vi "EndevoGOOP400Provider_Configuration.vi"(1 "ClassRef/ClassPath(If empty Configuration default will be modified)":variant, 5 "Error In":errorcluster) -> (15 "SelectedWireStyleIndex":i32, 19 "Error Out":errorcluster)   [LabVIEW 2020]
uses:
  <resource>/Framework/Providers/Open_GDS/ClassProviders/Common/LvIcon_class/GDSLvIcon_ColorControl.ctl
  <resource>/Framework/Providers/Open_GDS/SubVIs/GOOP_WirePattern.ctl
  <resource>/Framework/Providers/Open_GDS/ClassProviders/Common/ScriptingFunctions/Scripting_ConnectorPanePatternType.ctl
  <resource>/Framework/Providers/Open_GDS/ClassProviders/Provider_BaseClassInterface/BaseProvider_SubVIs/BaseProvider_WireStyleType.ctl
  <resource>/Framework/Providers/Open_GDS/SubVIs/GOOP_WireConfigurationType.ctl
  <resource>/Framework/Providers/Open_GDS/ClassProviders/Common/CommonVIs/CommonVIs_ClassIconSelection_Action.ctl
  <resource>/Framework/Providers/Open_GDS/ClassProviders/Provider_BaseClassInterface/BaseProvider_SubVIs/BaseProvider_FileNamingOption.ctl
  <resource>/Framework/Providers/Open_GDS/ClassProviders/Provider_EndevoGOOP400/GOOP400_SubVIs/GOOP400_Options.ctl
panel:
  in  "_CleanUpBDForPropertyMethods":bool caption="Use flat folder structure for new classes"
  in  "File naming option":T1(ring)
  out "IconSelection":picture
  in  "_FlatFolderStructure":bool caption="Use flat folder structure for new classes"
  in  "WireStyleList":T2[](array[typedef])
  in  "DiscardChanges":bool
  in  "Update/AddWireStyle":bool
  in  "DeleteWireStyle":bool
  in  "Down":bool
  in  "Up":bool
  in  "WireStyleName":string caption="Selected Wire Style Name"
  out "ProductPicture":picture
  out "Icon":picture
  in  "_Dice":cluster{"Boolean 2":bool, "Dice 2":bool}
  in  "_DefaultConnectorPanePattern":T3 caption="Default Connector Pane Pattern" items=["4x4x4", "5x6x5", "6x8x6"]
  in  "_HelpDefaultConfiguration":bool
  in  "_Help":bool
  out "_ClassItemIconApperance":string caption="Class Item Icon Appearance"
  out "_WireApperance":string
  in  "_SetToDefaultForAllClasses":bool caption="Set this to default\nfor all future classes"
  in  "_Cancel":bool
  out "_Preview":picture caption="Preview"
  in  "_Icon":u16(ring) caption="Icon" items=["BlueFull", "BlueFrame", "InterfaceBlue", "BlueCircle", "BrownFull", "BrownFrame", "InterfaceBrown", "BrownCircle", "BurgundyFull", "BurgundyFrame", "InterfaceBurgundy", "BurgundyCircle", "CyanFull", "CyanFrame", "InterfaceCyan", "CyanCircle", "DarkBlueFull", "DarkBlueFrame", "InterfaceDarkBlue", "DarkBlueCircle", "ForestGreenFull", "ForestGreenFrame", "InterfaceForestGreen", "ForestGreenCircle", "GrayFull", "GrayFrame", "InterfaceGray", "GrayCircle", "GreenFull", "GreenFrame", "InterfaceGreen", "GreenCircle", "LightGreenFull", "LightGreenFrame", "InterfaceLightGreen", "LightGreenCircle", "LightRedFull", "LightRedFrame", "InterfaceLightRed", "LightRedCircle", "PinkFull", "PinkFrame", "InterfacePink", "PinkCircle", "PurpleFull", "PurpleFrame", "InterfacePurple", "PurpleCircle", "RedFull", "RedFrame", "InterfaceRed", "RedCircle", "YellowFull", "YellowFrame", "InterfaceYellow", "YellowCircle"]
  in  "_TunnelsAndTerminalsColors":T4 caption="Tunnels and \nTerminals Colors"
  in  "_CenterColor2":T4 caption="Pattern Colors"
  in  "_CenterColor1":T4 caption="Pattern Colors"
  in  "_CenterPattern":T5 caption="Center pattern"
  in  "_EdgeColor":T4 caption="Edge color"
  in  "_CenterThickness":T6(ring) caption="Center thickness"
  in  "_EdgeThickness":T7(ring) caption="Edge thickness"
  out "Wire preview":picture
  in  "_Done":bool
  # "Wire Configuration"
  # "Wire Appearance"
  # "GOOP4 Options"
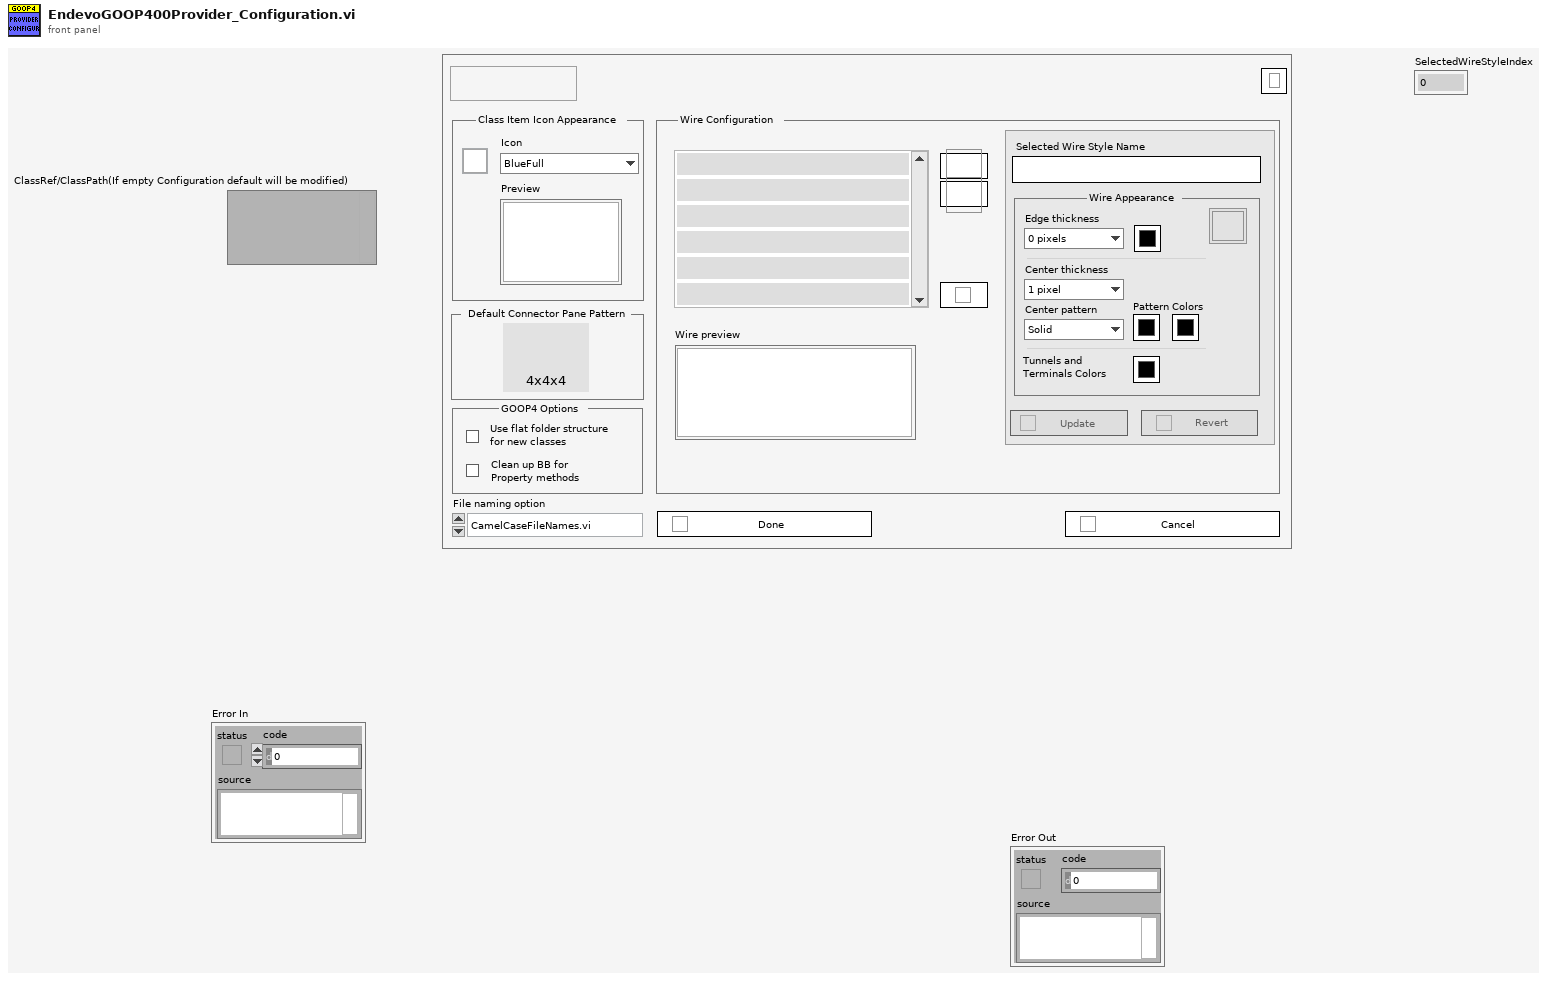
[diagram p1: front panel]
types:
  T1 = enum16{"CamelCaseFileNames.vi", "File Names With Spaces.vi", "File_Names_With_Underscores"}
  T2 = typedef "BaseProvider_WireStyleType.ctl" = cluster{"Boolean":bool, "Wire":picture, "Name":string, "Status":u16}
  T3 = typedef "Scripting_ConnectorPanePatternType.ctl" = u16
  T4 = typedef "GDSLvIcon_ColorControl.ctl" = cluster{"Decal":bool, "Color":u32}
  T5 = typedef "GOOP_WirePattern.ctl" = enum16{"Solid", "Large dash", "Small dash"}
  T6 = enum16{"1 pixel", "2 pixels", "3 pixels", "4 pixels", "5 pixels"}
  T7 = enum16{"0 pixels", "1 pixel", "2 pixels", "3 pixels"}
  T8 = typedef "GOOP_WireConfigurationType.ctl" = cluster{"Edge thickness":i32, "Edge color":u32, "Center thickness":i32, "Center pattern":T5, "CenterColor1":u32, "CenterColor2":u32, "Tunnels and terminals colors":u32}
  T9 = cluster{"FirstTime":bool, "ClassRef":refnum<vi>, "ClassRefCreated":bool, "CurrentWireStyle":T8, "DefaultIndex":i32, "SelectedWireStyleIndex":i32, "StartWireStyleIndex":i32}
  T10 = typedef "GOOP400_Options.ctl" = cluster{"FlatFolderStructure":bool, "CleanUpBDForPropertyMethods":bool}
  T11 = typedef "BaseProvider_FileNamingOption.ctl" = enum16{"CamelCase", "Space", "Underscore"}
  T12 = typedef "BaseProvider_IniFileSettings.ctl" = cluster{"ClassFolderSuffix":string, "InterfaceFolderSuffix":string, "InterfaceIcon":string, "FileNamingOption":T11, "DynamicDispatchStartValue":bool, "UseGetSetForPropertyNodeMethods":bool}
  T13 = typedef "GDSLvCLass_ClassSettingsType.ctl" = cluster{"ClassProviderName":string, "ClassTemplateUsed":string, "ClassTemplateVersion":string, "ClassDescription":string, "PlugIns":T14[], "ConnectorPanePattern":string}
  T14 = typedef "GDSLvClass_PlugIn.ctl" = cluster{"Type":T15, "ID":string, "Version":string, "Path":path, "Name":string, "Data":variant}
  T15 = typedef "GDSLvClass_PlugInTypes.ctl" = enum16{"DesignPattern", "MethodTypes"}
  T16 = cluster{"Foreground Color":u32, "Background Color":u32, "Fill Pattern":cluster{"Row 0":u8, "Row 1":u8, "Row 2":u8, "Row 3":u8, "Row 4":u8, "Row 5":u8, "Row 6":u8, "Row 7":u8}, "Width":i16, "Mode":enum16{"Copy", "Or", "Exclusive Or", "Bit Clear", "Not Copy", "Not Or", "Nor Exclusive Or", "Not Bit Clear"}, "Style":enum32{"Solid", "Dash", "Dot", "Dash Dot", "Dash Dot Dot"}, "Fill Rule":enum32{"Even Odd", "Winding"}, "End Caps":enum32{"Default", "Flat"}}[]
  T17 = enum8{"Enabled", "Disabled", "Disabled and Grayed Out"}
  T18 = typedef "imagedata.ctl" = cluster{"image type":i32, "image depth":i32, "image":u8[], "mask":u8[], "colors":u32[], "Rectangle":cluster{"left":i16, "top":i16, "right":i16, "bottom":i16}}
  T19 = typedef "CommonVIs_ClassIconSelection_Action.ctl" = enum16{"All", "Non Interface", "Only Interface"}
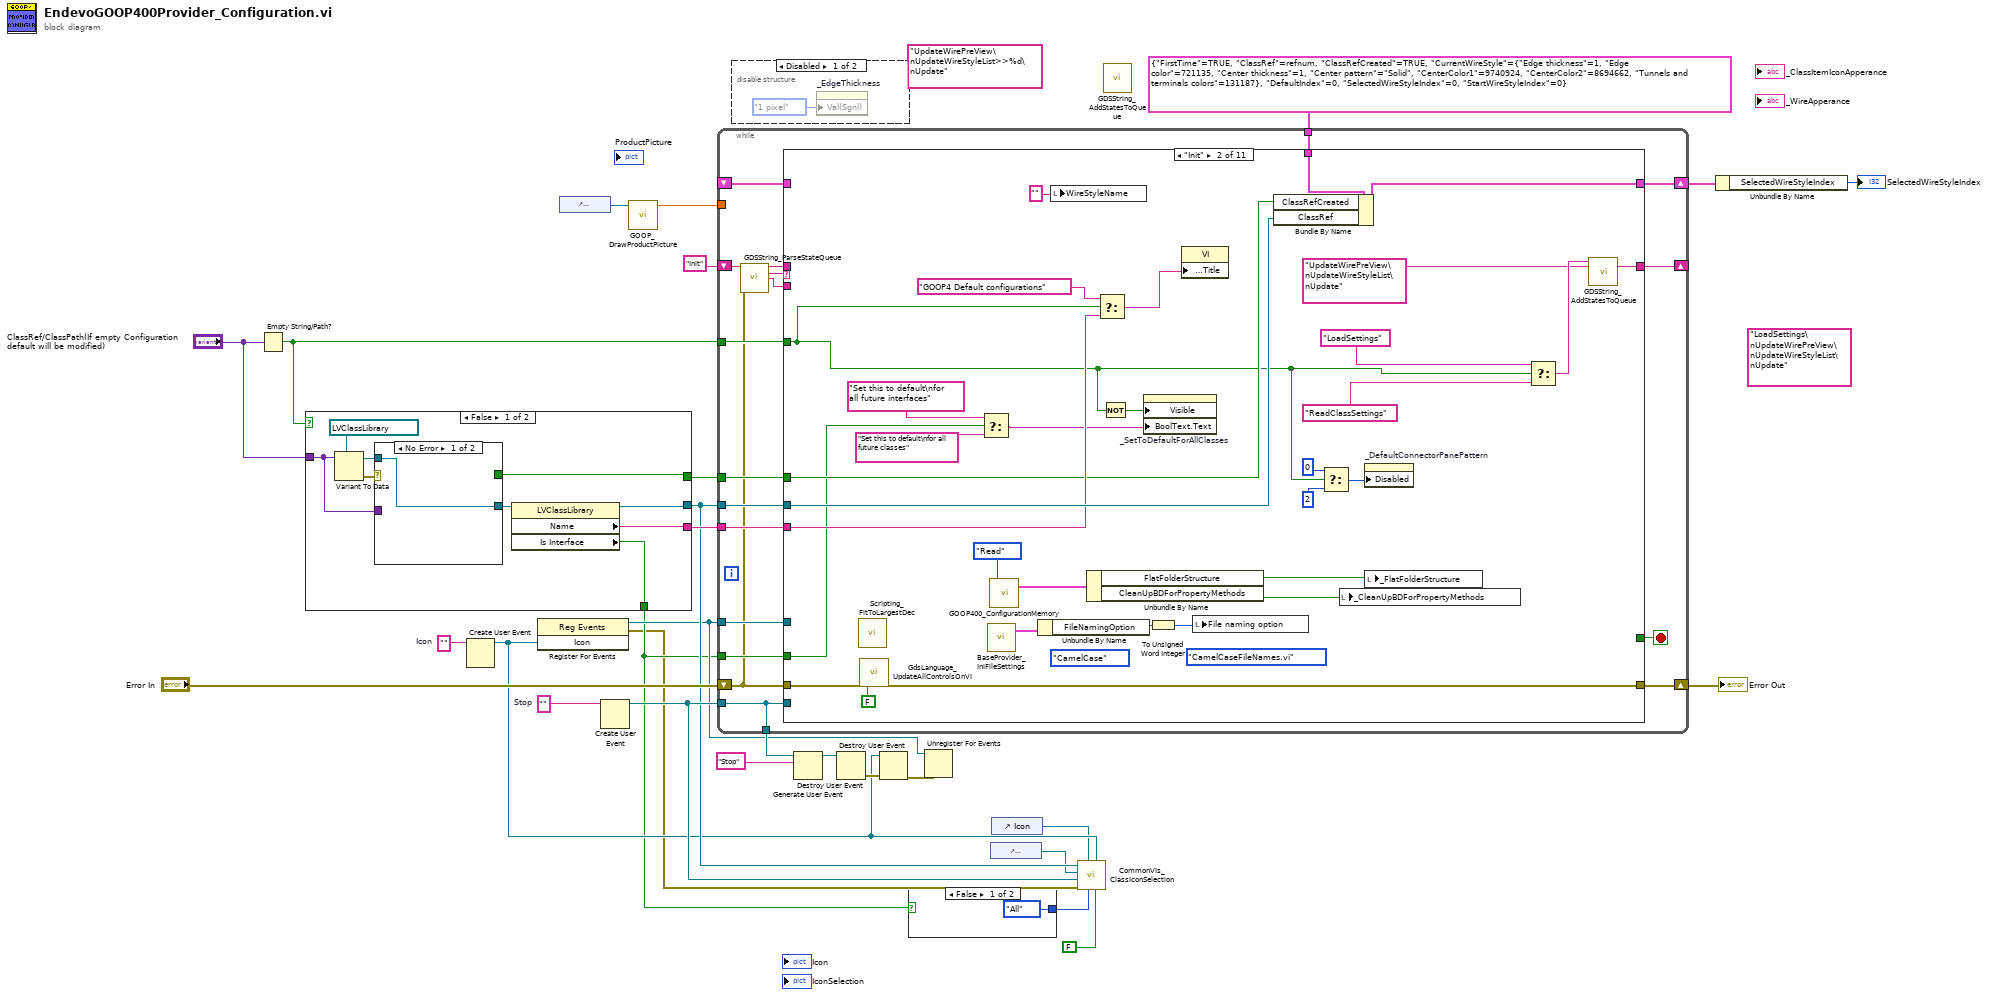
[diagram p0: block diagram]
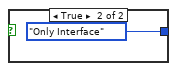
[diagram p2: hidden frame]
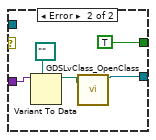
[diagram p4: hidden frame]
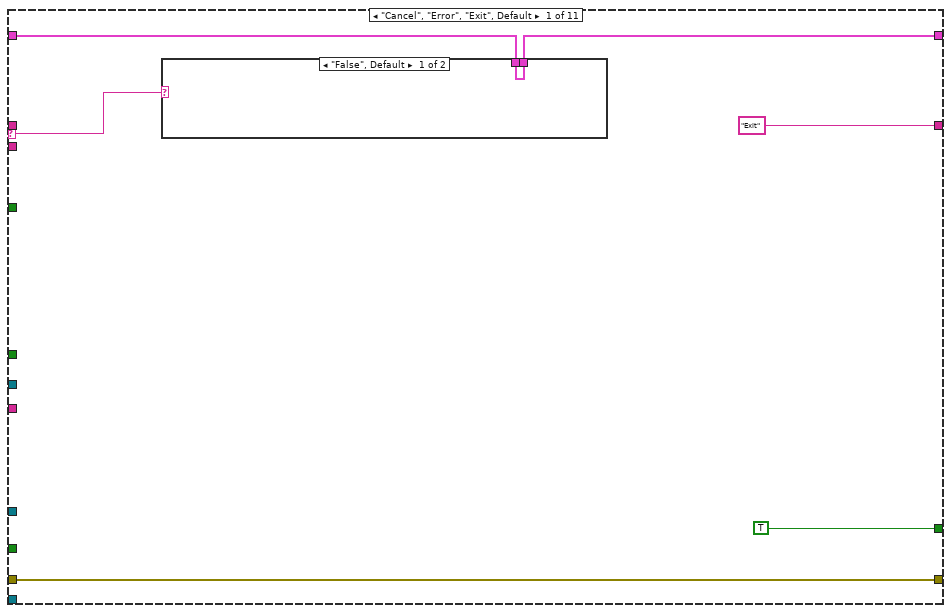
[diagram p6: hidden frame]
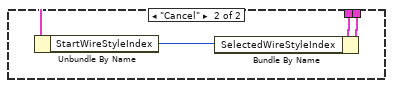
[diagram p7: hidden frame]
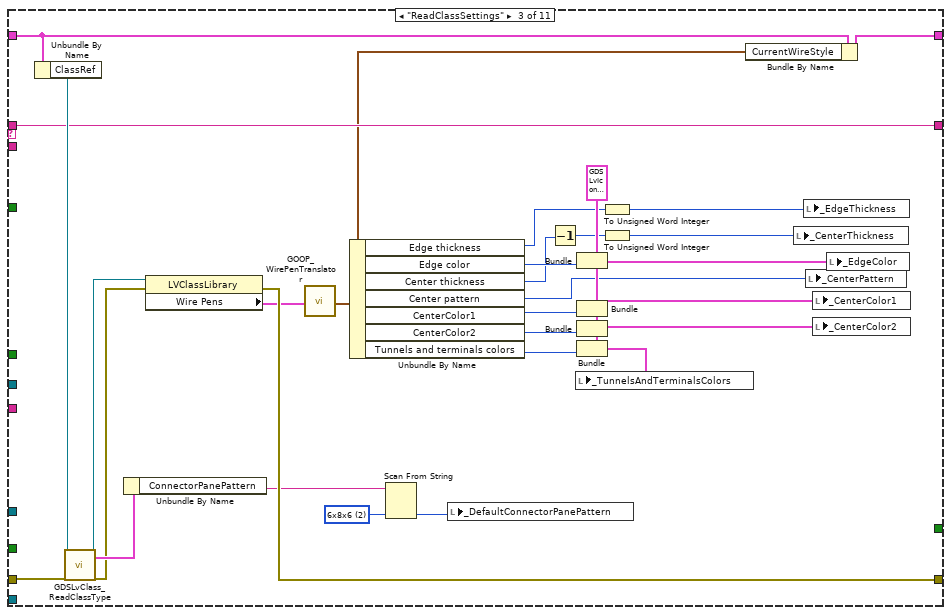
[diagram p8: hidden frame]
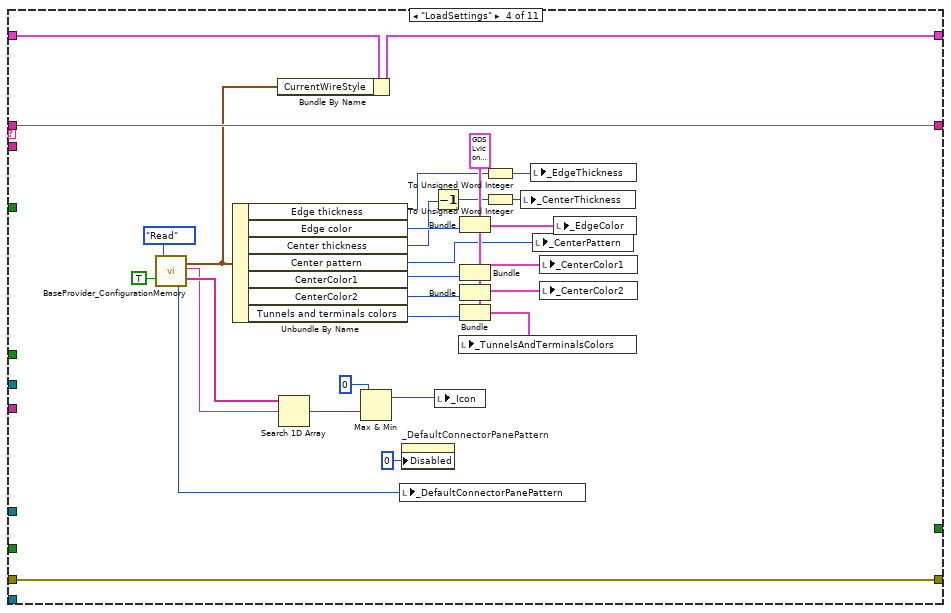
[diagram p9: hidden frame]
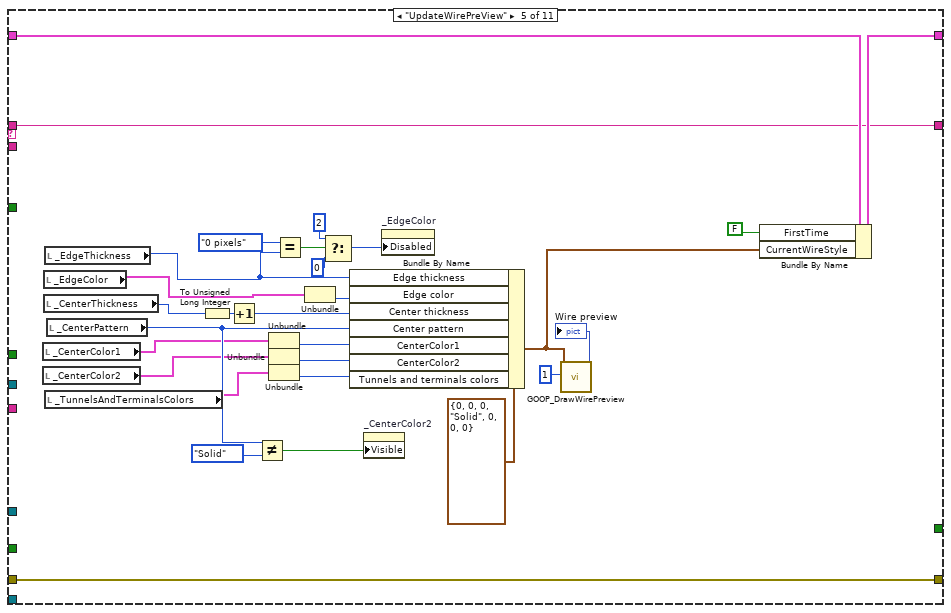
[diagram p10: hidden frame]
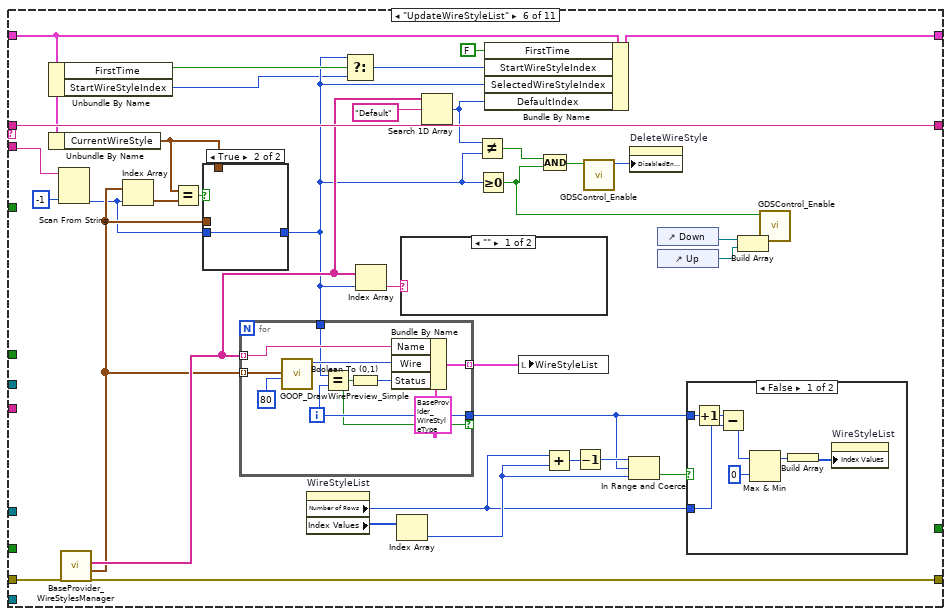
[diagram p11: hidden frame]
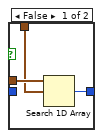
[diagram p12: hidden frame]
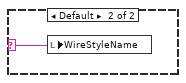
[diagram p14: hidden frame]
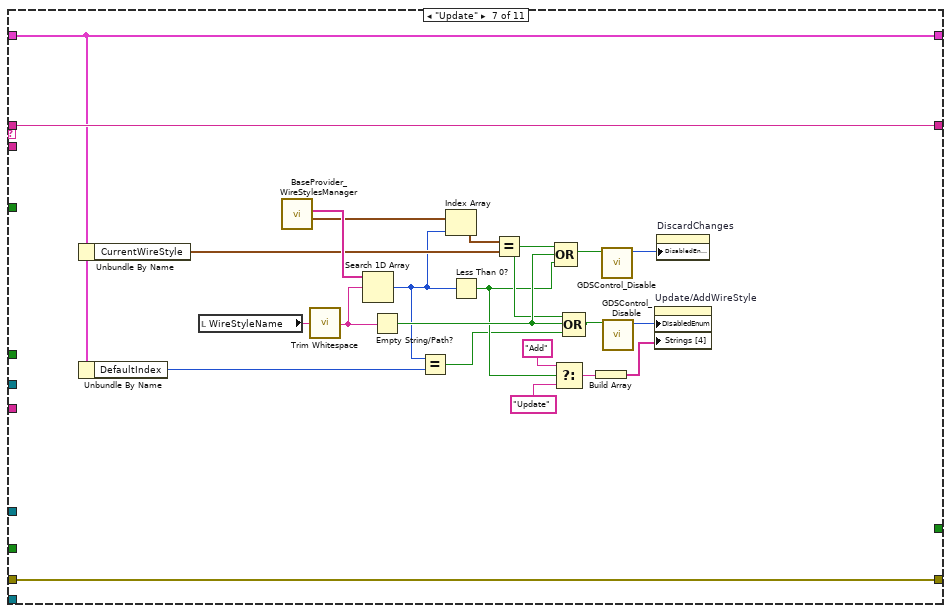
[diagram p15: hidden frame]
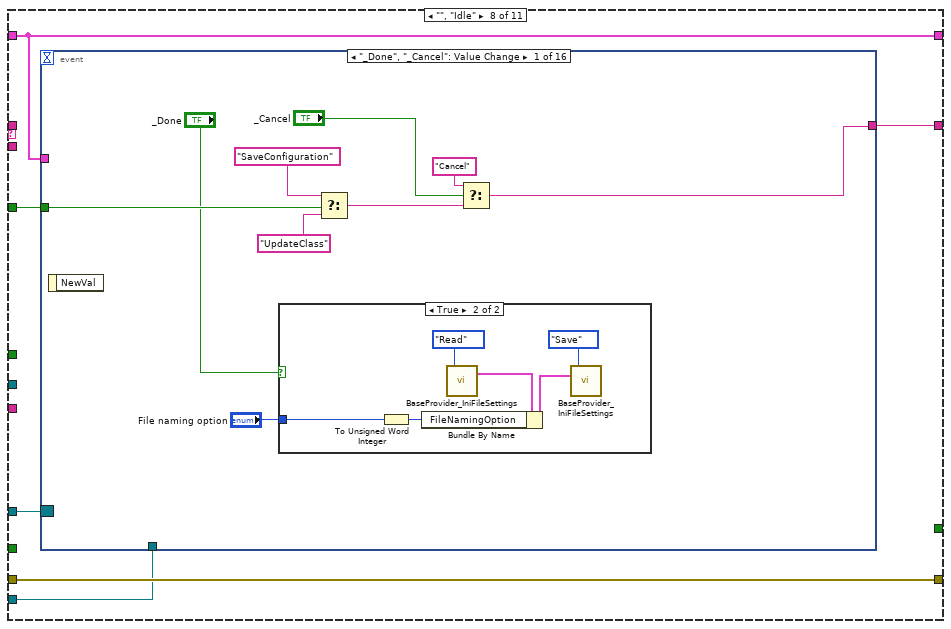
[diagram p16: hidden frame]
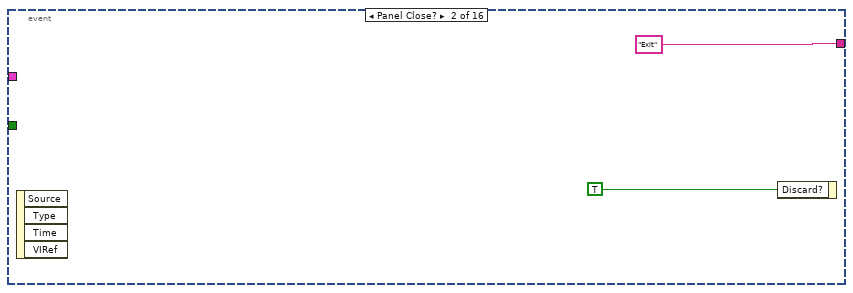
[diagram p18: hidden frame]
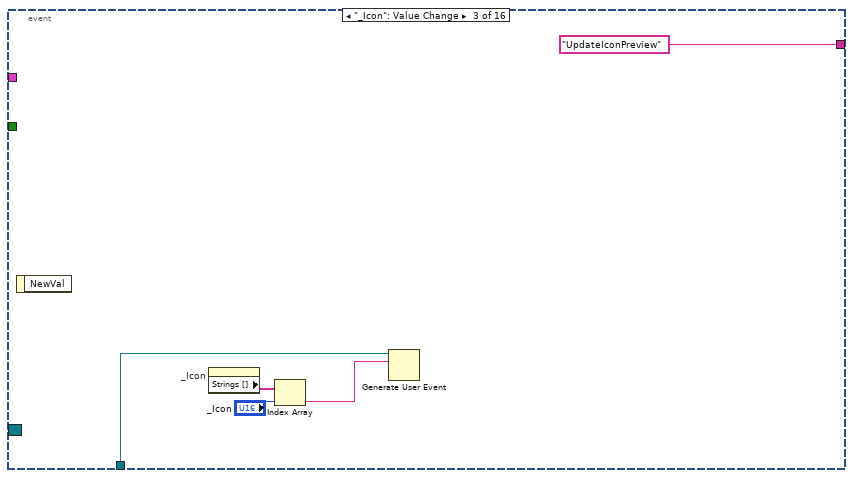
[diagram p19: hidden frame]
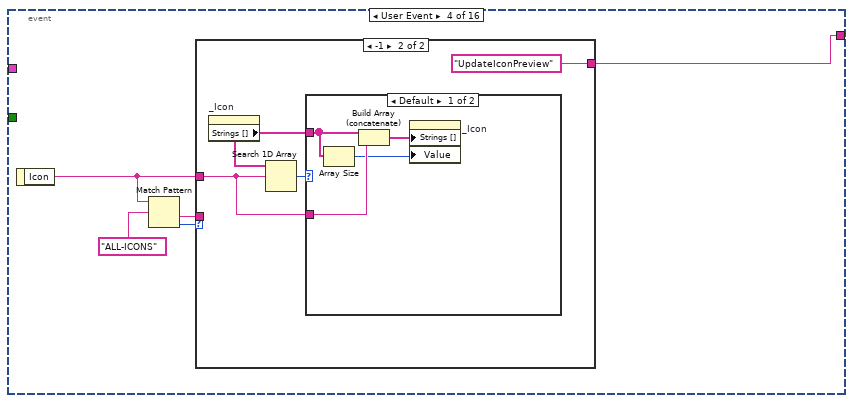
[diagram p20: hidden frame]
diagram:
  (unwired) "LoadSettings\nUpdateWirePreView\nUpdateWireStyleList\nUpdate"
  (unwired) "UpdateWirePreView\nUpdateWireStyleList>>%d\nUpdate"
  w16 = ""  # Icon
  w19 = ""  # Stop
  n1 = Empty String/Path?(string/path="ClassRef/ClassPath(If empty Configuration default will be modified)") -> (empty?=w21:bool)
  n2 = case shown="False" w21 {
    tunnel: "ClassRef/ClassPath(If empty Configuration default will be modified)" -> [w36 _]
    tunnel: [w32 _] -> w17
    tunnel: [w34 _] -> w24
    tunnel: [w31 _] -> w23
    tunnel: [w30 _] -> w11
    frame False {
      n3 = Variant To Data(type=refnum<vi> refnum ("Class Refnum In"), Variant=w36) -> (data=w35:refnum<vi>, error out=w37:errorcluster)  [unwired: 1 in]
      n4 = case shown="No Error" w37 {
        tunnel: w36 -> [_ w44]
        tunnel: [w39 w41] -> w33
        tunnel: w35 -> [w39 _]
        tunnel: [_ TRUE] -> w34
        frame No Error {
        }
        frame Error {
          n5 = Variant To Data(type=path "", Variant=w44) -> (data=w42:path)  [unwired: 1 in, 1 out]
          n6 = call <resource>:"GDSLvClass_OpenClass.vi"("ClassToOpen"=w42) -> ("LVClass.Open"=w41:refnum<vi>)  [unwired: 17 in, 1 out]
        }
      }
      n7 = property class="LVClassLibrary"(reference=w33) -> (reference out=w32:refnum<vi>, "Name"=w31:string, "Is Interface"=w30:bool)  [unwired: 1 in, 1 out]
    }
    frame True {
    }
  }
  n8 = Create User Event(user event datatype=w16) -> (user event=w12:refnum<user-event>)  [unwired: 1 in, 1 out]
  n9 = register-events(w12) -> (reference out=w15:refnum<event-registration>, error out=w10:errorcluster)  [unwired: 2 in]
  n10 = control-ref of="ProductPicture"() -> (w9:refnum<vi>)
  n11 = Create User Event(user event datatype=w19) -> (user event=w20:refnum<user-event>)  [unwired: 1 in, 1 out]
  n12 = call <resource>:"GOOP_DrawProductPicture.vi"("ProductPictureControl"=w9) -> ("Zoom Factor"=w8:sgl)  [unwired: 10 in]
  n13 = while {
    shift-right: [w62] -> w27
    shift-left: "Error In" -> [w51]
    shift-right: [w47] -> _
    shift-left: "Init" -> [w52]
    shift-right: [w61] -> w6
    shift-left: _ -> [w60]
    tunnel: w20 -> [w55]
    tunnel: [w55] -> w25
    tunnel: w21 -> [w59]
    tunnel: w17 -> [w58]
    tunnel: w24 -> [w57]
    tunnel: w23 -> [w56]
    tunnel: w15 -> [w54]
    tunnel: w11 -> [w53]
    tunnel: w8 -> [_]
    tunnel: T9 {"FirstTime"=TRUE, "ClassRef"=refnum, "ClassRefCreated"=TRUE, "CurrentWireStyle"={"Edge thickness"=1, "Edge color"=721135, "Center thickness"=1, "Center pattern"=enum."Solid", "CenterColor1"=9740924, "CenterColor2"=8694662, "Tunnels and terminals colors"=131187}, "DefaultIndex"=0, "SelectedWireStyleIndex"=0, "StartWireStyleIndex"=0} -> [w45]
    stop <- w46 stop-if-true
    n14 = call <resource>:"GDSString_ParseStateQueue.vi"("State Queue"=w52, "Error In (no error)"=w51) -> ("Remaining States"=w49:string, "Current State"=w50:string, "Arguments"=w48:string)  [unwired: 9 in, 2 out]
    n15 = case shown="\"Init\"" w50 {
      selector: w50 -> [w63 _ _ _ _ _ _ _ _ _ _]
      tunnel: w51 -> [w68 w99 w115 w147 w169 w227 w262 w277 w437 w491 w517]
      tunnel: [w68 w98 w132 w147 w169 w224 w262 w277 w443 w491 w517] -> w62
      tunnel: ["Exit" w83 w108 w137 w163 w226 w272 w278 w470 "Idle" "Exit"] -> w47
      tunnel: [w65 w101 w107 w135 w168 w213 w253 w273 w465 w492 w501] -> w61
      tunnel: w60 -> [w64 _ w133 w134 w164 w196 w253 w273 w465 w492 w515]
      tunnel: w59 -> [_ w89 _ _ _ _ _ w276 _ _ _]
      tunnel: w58 -> [_ w96 _ _ _ _ _ _ _ _ _]
      tunnel: w57 -> [_ w94 _ _ _ _ _ _ _ _ _]
      tunnel: w56 -> [_ w95 _ _ _ _ _ _ _ _ _]
      tunnel: w55 -> [_ _ _ _ _ _ _ w274 _ _ _]
      tunnel: w54 -> [_ _ _ _ _ _ _ w275 _ _ _]
      tunnel: w53 -> [_ w93 _ _ _ _ _ _ _ _ w512]
      tunnel: w49 -> [_ _ w108 w137 w163 w226 w272 _ _ _ _]
      tunnel: w48 -> [_ _ _ _ _ w203 _ _ _ _ _]
      tunnel: [TRUE _ _ _ _ _ _ _ _ _ _] -> w46
      tunnel: w45 -> [_ w82 _ _ _ _ _ _ _ _ _]
      frame "Cancel", "Error", "Exit", Default {
        n16 = case shown="\"False\", Default" w63 {
          tunnel: [w69 w72] -> w65
          tunnel: w64 -> [w69 w71]
          frame "False", Default {
          }
          frame "Cancel" {
            n17 = Unbundle By Name(w71) -> ("StartWireStyleIndex"=w70:i32)
            n18 = Bundle By Name(cluster=w71, "SelectedWireStyleIndex"=w70) -> (w72:T9)
          }
        }
      }
      frame "Init" {
        (unwired) T1."CamelCaseFileNames.vi" ("File naming option")
        (unwired) BaseProvider_FileNamingOption."CamelCase" ("FileNamingOption")
        n19 = call <resource>:"Scripting_FitToLargestDec.vi"() -> ()  [unwired: 6 in, 2 out]
        n20 = call <resource>:"GdsLanguage_UpdateAllControlsOnVI.vi"("error in (no error)"=w99, "CreateLanguageFile(Use this to create a languageFile)"=FALSE) -> ("error out"=w98:errorcluster)  [unwired: 16 in, 1 out]
        n21 = Select(t="Set this to default\nfor all future interfaces", s=w93, f="Set this to default\nfor all future classes") -> (s? t:f=w90:string)
        n22 = call <resource>:"BaseProvider_IniFileSettings.vi"() -> ("IniFileSettings"=w76:T12)  [unwired: 18 in, 1 out]
        n23 = call <resource>:"GOOP400_ConfigurationMemory.vi"("Action"=enum16{"Read", "Load", "Save"}."Read") -> ("OptionsOut"=w79:T10)  [unwired: 17 in, 1 out]
        n24 = Unbundle By Name(w76) -> ("FileNamingOption"=w75:T11)
        n25 = local write "WireStyleName"("" ("WireStyleName")) -> ()
        n26 = Unbundle By Name(w79) -> ("FlatFolderStructure"=w77:bool, "CleanUpBDForPropertyMethods"=w73:bool)
        n27 = Select(t="GOOP4 Default configurations", s=w89, f=w95) -> (s? t:f=w80:string)
        n28 = Not(x=w89) -> (.not. x?=w100:bool)
        n29 = property on="_SetToDefaultForAllClasses" class="Bool (strict)"("Visible"=w100, "BoolText.Text"=w90) -> ()  [unwired: 2 in, 2 out]
        n30 = To Unsigned Word Integer(number=w75) -> (unsigned 16bit integer=w74:u16)
        n31 = property class="VI"("Front Panel.Title"=w80) -> ()  [unwired: 2 in, 2 out]
        n32 = local write "File naming option"(w74) -> ()
        n33 = Bundle By Name(cluster=w82, "ClassRefCreated"=w94, "ClassRef"=w96) -> (w101:T9)
        n34 = Select(t=u8 0 ("Disabled"), s=w89, f=u8 2 ("Disabled")) -> (s? t:f=w87:u8)
        n35 = local write "_CleanUpBDForPropertyMethods"(w73) -> ()
        n36 = property on="_DefaultConnectorPanePattern" class="Ring (strict)"("Disabled"=w87) -> ()  [unwired: 2 in, 2 out]
        n37 = local write "_FlatFolderStructure"(w77) -> ()
        n38 = Select(t="LoadSettings", s=w89, f="ReadClassSettings") -> (s? t:f=w85:string)
        n39 = call <resource>:"GDSString_AddStatesToQueue.vi"("State(s) in Front (\"\")"=w85, "State(s) in (\"\")"="UpdateWirePreView\nUpdateWireStyleList\nUpdate") -> ("States Out"=w83:string)  [unwired: 13 in]
      }
      frame "ReadClassSettings" {
        w112 = T3 2 items=["4x4x4", "5x6x5", "6x8x6"] ("Pattern")
        w125 = T4 {"Decal"=FALSE, "Color"=11184810} ("Edge color")
        n40 = Unbundle By Name(w133) -> ("ClassRef"=w114:refnum<vi>)
        n41 = call <resource>:"GDSLvClass_ReadClassType.vi"("Class Refnum In"=w114, "error in (no error)"=w115) -> ("Class Refnum Out"=w109:refnum<vi>, "ClassSettings"=w113:T13, "error out"=w105:errorcluster)  [unwired: 15 in]
        n42 = Unbundle By Name(w113) -> ("ConnectorPanePattern"=w111:string)
        n43 = property class="LVClassLibrary"(reference=w109, error in=w105) -> (error out=w132:errorcluster, "Wire Pens"=w131:T16)  [unwired: 1 out]
        n44 = call <resource>:"GOOP_WirePenTranslator.vi"("WirePensIn"=w131) -> ("WireConfigurationOut"=w106:T8)  [unwired: 17 in, 1 out]
        n45 = Unbundle By Name(w106) -> ("Edge thickness"=w117:i32, "Edge color"=w130:u32, "Center thickness"=w120:i32, "Center pattern"=w121:T5, "CenterColor1"=w129:u32, "CenterColor2"=w128:u32, "Tunnels and terminals colors"=w127:u32)
        n46 = Scan From String(input string=w111, default 1=w112) -> (output 1=w110:T3)  [unwired: 3 in, 3 out]
        n47 = local write "_DefaultConnectorPanePattern"(w110) -> ()
        n48 = Decrement(x=w120) -> (x-1=w119:i32)
        n49 = Bundle(cluster=w125, "Color"=w130) -> (w122:T4)  [unwired: 1 in]
        n50 = Bundle(cluster=w125, "Color"=w129) -> (w123:T4)  [unwired: 1 in]
        n51 = Bundle(cluster=w125, "Color"=w128) -> (w124:T4)  [unwired: 1 in]
        n52 = Bundle(cluster=w125, "Color"=w127) -> (w126:T4)  [unwired: 1 in]
        n53 = local write "_TunnelsAndTerminalsColors"(w126) -> ()
        n54 = To Unsigned Word Integer(number=w117) -> (unsigned 16bit integer=w116:u16)
        n55 = To Unsigned Word Integer(number=w119) -> (unsigned 16bit integer=w118:u16)
        n56 = Bundle By Name(cluster=w133, "CurrentWireStyle"=w106) -> (w107:T9)
        n57 = local write "_CenterThickness"(w118) -> ()
        n58 = local write "_EdgeThickness"(w116) -> ()
        n59 = local write "_CenterPattern"(w121) -> ()
        n60 = local write "_CenterColor1"(w123) -> ()
        n61 = local write "_CenterColor2"(w124) -> ()
        n62 = local write "_EdgeColor"(w122) -> ()
      }
      frame "LoadSettings" {
        w157 = T4 {"Decal"=FALSE, "Color"=11184810} ("Edge color")
        n63 = call <resource>:"BaseProvider_ConfigurationMemory.vi"("Filter_Icons"=TRUE, "Action"=enum16{"Read", "Load", "Save"}."Read") -> ("PatternOut"=w140:T3, "WireConfigurationOut"=w136:T8, "IconOut"=w144:string, "ClassItemIconNames"=w145:string[])  [unwired: 11 in, 3 out]
        n64 = Unbundle By Name(w136) -> ("Edge thickness"=w149:i32, "Edge color"=w162:u32, "Center thickness"=w152:i32, "Center pattern"=w153:T5, "CenterColor1"=w161:u32, "CenterColor2"=w160:u32, "Tunnels and terminals colors"=w159:u32)
        n65 = Bundle By Name(cluster=w134, "CurrentWireStyle"=w136) -> (w135:T9)
        n66 = Search 1D Array(1D array=w145, element=w144) -> (index of element=w142:i32)  [unwired: 1 in]
        n67 = Max & Min(x=0, y=w142) -> (max(x,y)=w141:i32)  [unwired: 1 out]
        n68 = local write "_DefaultConnectorPanePattern"(w140) -> ()
        n69 = property on="_DefaultConnectorPanePattern" class="Ring (strict)"("Disabled"=u8 0) -> ()  [unwired: 2 in, 2 out]
        n70 = Decrement(x=w152) -> (x-1=w151:i32)
        n71 = local write "_Icon"(w141) -> ()
        n72 = Bundle(cluster=w157, "Color"=w162) -> (w154:T4)  [unwired: 1 in]
        n73 = Bundle(cluster=w157, "Color"=w161) -> (w155:T4)  [unwired: 1 in]
        n74 = Bundle(cluster=w157, "Color"=w160) -> (w156:T4)  [unwired: 1 in]
        n75 = Bundle(cluster=w157, "Color"=w159) -> (w158:T4)  [unwired: 1 in]
        n76 = local write "_TunnelsAndTerminalsColors"(w158) -> ()
        n77 = To Unsigned Word Integer(number=w149) -> (unsigned 16bit integer=w148:u16)
        n78 = To Unsigned Word Integer(number=w151) -> (unsigned 16bit integer=w150:u16)
        n79 = local write "_CenterThickness"(w150) -> ()
        n80 = local write "_EdgeThickness"(w148) -> ()
        n81 = local write "_CenterPattern"(w153) -> ()
        n82 = local write "_CenterColor1"(w155) -> ()
        n83 = local write "_CenterColor2"(w156) -> ()
        n84 = local write "_EdgeColor"(w154) -> ()
      }
      frame "UpdateWirePreView" {
        n85 = local read "_CenterColor1"() -> (w172:T4)
        n86 = local read "_CenterColor2"() -> (w171:T4)
        n87 = local read "_EdgeColor"() -> (w175:T4)
        n88 = local read "_CenterThickness"() -> (w174:T6)
        n89 = local read "_EdgeThickness"() -> (w176:T7)
        n90 = local read "_TunnelsAndTerminalsColors"() -> (w170:T4)
        n91 = local read "_CenterPattern"() -> (w173:T5)
        n92 = To Unsigned Long Integer(number=w174) -> (unsigned 32bit integer=w191:u32)
        n93 = Increment(x=w191) -> (x+1=w184:u32)
        n94 = Not Equal?(x=w173, y=GOOP_WirePattern."Solid") -> (x != y?=w166:bool)
        n95 = Unbundle(w172) -> ("Color"=w182:u32)  [unwired: 1 out]
        n96 = Unbundle(w171) -> ("Color"=w183:u32)  [unwired: 1 out]
        n97 = Unbundle(w170) -> ("Color"=w180:u32)  [unwired: 1 out]
        n98 = Equal?(x=T7."0 pixels", y=w176) -> (x = y?=w186:bool)
        n99 = Unbundle(w175) -> ("Color"=w181:u32)  [unwired: 1 out]
        n100 = Select(t=u8 2 ("Disabled"), s=w186, f=u8 0) -> (s? t:f=w188:u8)
        n101 = Bundle By Name(cluster=T8 {"Edge thickness"=0, "Edge color"=0, "Center thickness"=0, "Center pattern"=enum."Solid", "CenterColor1"=0, "CenterColor2"=0, "Tunnels and terminals colors"=0} ("WireConfiguration"), "Edge thickness"=w176, "Edge color"=w181, "Center thickness"=w184, "Center pattern"=w173, "CenterColor1"=w182, "CenterColor2"=w183, "Tunnels and terminals colors"=w180) -> (w165:T8)
        n102 = property on="_CenterColor2" class="Clust (strict)"("Visible"=w166) -> ()  [unwired: 2 in, 2 out]
        n103 = property on="_EdgeColor" class="Clust (strict)"("Disabled"=w188) -> ()  [unwired: 2 in, 2 out]
        n104 = call <resource>:"GOOP_DrawWirePreview.vi"("WireConfiguration"=w165, "Zoom"=1) -> ("Picture"=→"Wire preview":picture)  [unwired: 16 in, 1 out]
        n105 = Bundle By Name(cluster=w164, "FirstTime"=FALSE, "CurrentWireStyle"=w165) -> (w168:T9)
      }
      frame "UpdateWireStyleList" {
        n106 = Unbundle By Name(w196) -> ("FirstTime"=w195:bool, "StartWireStyleIndex"=w192:i32)
        n107 = Unbundle By Name(w196) -> ("CurrentWireStyle"=w201:T8)
        n108 = Scan From String(input string=w203, default 1=-1 ("default value 1")) -> (output 1=w198:i32)  [unwired: 3 in, 3 out]
        n109 = call <resource>:"BaseProvider_WireStylesManager.vi"("error in (no error)"=w227) -> ("error out"=w224:errorcluster, "AllWireConfigurations"=w204:T8[], "AllWireConfigurations(Names)"=w215:string[])  [unwired: 7 in, 1 out]
        n110 = Index Array(array=w204, index=w198) -> (element=w200:T8)
        n111 = Equal?(x=w201, y=w200) -> (x = y?=w199:bool)
        n112 = case shown="True" w199 {
          tunnel: [w230 w231] -> w194
          tunnel: w204 -> [w229 _]
          tunnel: w201 -> [w228 _]
          tunnel: w198 -> [_ w231]
          frame False {
            n113 = Search 1D Array(1D array=w229, element=w228) -> (index of element=w230:i32)  [unwired: 1 in]
          }
          frame True {
          }
        }
        n114 = for {
          tunnel: w215 -> [w245] mode=indexing
          tunnel: w204 -> [w248] mode=indexing
          tunnel: [w244] -> w225 mode=indexing
          tunnel: w194 -> [w243]
          tunnel: [w241] -> w217 if=w240
          i -> [w241]
          n115 = call <resource>:"GOOP_DrawWirePreview_Simple.vi"("WireLength(100px)"=i16 80, "WireConfiguration"=w248) -> ("WirePictureOut"=w246:picture)  [unwired: 5 in, 4 out]
          n116 = Equal?(x=w243, y=w241) -> (x = y?=w240:bool)
          n117 = Boolean To (0,1)(Boolean=w240) -> (0, 1=w242:i16)
          n118 = Bundle By Name(cluster=T2 {"Boolean"=FALSE, "Wire"=bytes[0], "Name"="", "Status"=0} ("Cluster 2"), "Name"=w245, "Wire"=w246, "Status"=w242) -> (w244:T2)
        }
        n119 = property on="WireStyleList" class="Arr (strict)"() -> ("Number of Rows"=w216:u32, "Index Values"=w222:u32[])  [unwired: 2 in, 2 out]
        n120 = Select(t=w194, s=w195, f=w192) -> (s? t:f=w193:i32)
        n121 = Index Array(array=w215, index=w194) -> (element=w223:string)
        n122 = Index Array(array=w222) -> (element=w221:u32)  [unwired: 1 in]
        n123 = case shown="\"\"" w223 {
          selector: w223 -> [_ w239]
          frame "" {
          }
          frame Default {
            n124 = local write "WireStyleName"(w239) -> ()
          }
        }
        n125 = Search 1D Array(1D array=w215, element="Default") -> (index of element=w212:i32)  [unwired: 1 in]
        n126 = Not Equal?(x=w212, y=w194) -> (x != y?=w211:bool)
        n127 = Greater Or Equal To 0?(x=w194) -> (x >= 0?=w208:bool)
        n128 = Bundle By Name(cluster=w196, "FirstTime"=FALSE, "StartWireStyleIndex"=w193, "SelectedWireStyleIndex"=w194, "DefaultIndex"=w212) -> (w213:T9)
        n129 = local write "WireStyleList"(w225) -> ()
        n130 = Compound Arithmetic op=AND(w211, w208) -> (w210:bool)
        n131 = Add(x=w216, y=w221) -> (x+y=w220:u32)
        n132 = Decrement(x=w220) -> (x-1=w219:u32)
        n133 = call <resource>:"GDSControl_Enable.vi"("Enable(True)"=w210) -> ("Enable Property"=w209:T17)  [unwired: 10 in]
        n134 = In Range and Coerce(upper limit=w219, x=w217, lower limit=w221) -> (In Range?=w218:bool)  [unwired: 1 out]
        n135 = property on="DeleteWireStyle" class="Bool"("DisabledEnum"=w209) -> ()  [unwired: 2 in, 2 out]
        n136 = control-ref of="Down"() -> (w207:refnum<vi>)
        n137 = control-ref of="Up"() -> (w206:refnum<vi>)
        n138 = case shown="False" w218 {
          tunnel: w217 -> [w237 _]
          tunnel: w216 -> [w236 _]
          frame False {
            n139 = Increment(x=w237) -> (x+1=w232:i32)
            n140 = Subtract(x=w232, y=w236) -> (x-y=w235:u32)
            n141 = Max & Min(x=w235, y=u32 0) -> (max(x,y)=w233:u32)  [unwired: 1 out]
            n142 = Build Array(w233) -> (w238:u32[])
            n143 = property on="WireStyleList" class="Arr (strict)"("Index Values"=w238) -> ()  [unwired: 2 in, 2 out]
          }
          frame True {
          }
        }
        n144 = Build Array(w207, w206) -> (w205:refnum<vi>[])
        n145 = call <resource>:"GDSControl_Enable.vi"("ManyControls"=w205, "Enable(True)"=w208) -> ()  [unwired: 9 in, 1 out]
      }
      frame "Update" {
        n146 = Unbundle By Name(w253) -> ("CurrentWireStyle"=w266:T8)
        n147 = Unbundle By Name(w253) -> ("DefaultIndex"=w251:i32)
        n148 = local read "WireStyleName"() -> (w271:string)
        n149 = call <resource>:"BaseProvider_WireStylesManager.vi"() -> ("AllWireConfigurations"=w267:T8[], "AllWireConfigurations(Names)"=w269:string[])  [unwired: 8 in, 2 out]
        n150 = call <vilib>:"Trim Whitespace.vi"("string"=w271) -> ("trimmed string"=w268:string)  [unwired: 1 in]
        n151 = Search 1D Array(1D array=w269, element=w268) -> (index of element=w252:i32)  [unwired: 1 in]
        n152 = Empty String/Path?(string/path=w268) -> (empty?=w261:bool)
        n153 = Equal?(x=w252, y=w251) -> (x = y?=w250:bool)
        n154 = Index Array(array=w267, index=w252) -> (element=w265:T8)
        n155 = Less Than 0?(x=w252) -> (x < 0?=w258:bool)
        n156 = Equal?(x=w265, y=w266) -> (x = y?=w259:bool)
        n157 = Select(t="Add", s=w258, f="Update") -> (s? t:f=w255:string)
        n158 = Compound Arithmetic op=OR(w259, w261, w258) -> (w264:bool)
        n159 = Compound Arithmetic op=OR(w259, w261, w250) -> (w260:bool)
        n160 = Build Array(w255) -> (w254:string[])
        n161 = call <resource>:"GDSControl_Disable.vi"("Disasble(True)"=w264) -> ("Enable Property"=w263:T17)  [unwired: 10 in]
        n162 = call <resource>:"GDSControl_Disable.vi"("Disasble(True)"=w260) -> ("Enable Property"=w270:T17)  [unwired: 10 in]
        n163 = property on="Update/AddWireStyle" class="Bool"("DisabledEnum"=w270, "Strings [4]"=w254) -> ()  [unwired: 2 in, 2 out]
        n164 = property on="DiscardChanges" class="Bool"("DisabledEnum"=w263) -> ()  [unwired: 2 in, 2 out]
      }
      frame "", "Idle" {
        n165 = event shown="[0] \"_Done\", \"_Cancel\": Value Change" {
          selector: w275 -> [_ _ _ _ _ _ _ _ _ _ _ _ _ _ _ _]
          dyn-events: _ -> [_ _ _ _ _ _ _ _ _ _ _ _ _ _ _ _]
          timeout: _ -> [_ _ _ _ _ _ _ _ _ _ _ _ _ _ _ _]
          tunnel: [w283 "Exit" "UpdateIconPreview" w301 "UpdateWirePreView\nUpdate" "Idle" "UpdateWirePreView\nUpdate" w332 "Update" w363 "UpdateWirePreView\nUpdateWireStyleList\nUpdate" "UpdateWirePreView\nUpdateWireStyleList\nUpdate" w408 "Idle" "Idle" "Idle"] -> w278
          tunnel: w276 -> [w281 _ _ _ _ _ _ _ _ _ _ _ _ _ _ _]
          tunnel: w274 -> [_ _ w298 _ _ _ _ _ _ _ _ _ _ _ _ _]
          tunnel: w273 -> [_ _ _ _ _ _ _ _ _ _ _ w403 w417 _ _ _]
          event "_Done", "_Cancel": Value Change {
            n166 = event-data() -> ()  [unwired: 1 in, 1 out]
            n167 = case shown="True" "_Done" {
              tunnel: "File naming option" -> [_ w288]
              frame False {
              }
              frame True {
                n168 = To Unsigned Word Integer(number=w288) -> (unsigned 16bit integer=w289:u16)
                n169 = call <resource>:"BaseProvider_IniFileSettings.vi"("Action"=enum16{"Read", "Load", "Save"}."Read") -> ("IniFileSettings"=w293:T12)  [unwired: 17 in, 1 out]
                n170 = Bundle By Name(cluster=w293, "FileNamingOption"=w289) -> (w290:T12)
                n171 = call <resource>:"BaseProvider_IniFileSettings.vi"("IniFileSettings"=w290, "Action"=enum16{"Read", "Load", "Save"}."Save") -> ()  [unwired: 16 in, 2 out]
              }
            }
            n172 = Select(t="SaveConfiguration", s=w281, f="UpdateClass") -> (s? t:f=w284:string)
            n173 = Select(t="Cancel", s="_Cancel", f=w284) -> (s? t:f=w283:string)
          }
          event Panel Close? {
            n174 = event-data() -> ()  [unwired: 1 in, 4 out]
            n175 = event-data("Discard?"=TRUE) -> ()  [unwired: 1 in, 1 out]
          }
          event "_Icon": Value Change {
            n176 = event-data() -> ()  [unwired: 1 in, 1 out]
            n177 = property on="_Icon" class="Ring (strict)"() -> ("Strings []"=w299:string[])  [unwired: 2 in, 2 out]
            n178 = Index Array(array=w299, index="_Icon") -> (element=w297:string)
            n179 = Generate User Event(user event=w298, event data cluster=w297) -> ()  [unwired: 2 in, 2 out]
          }
          event User Event {
            n180 = event-data() -> ("Icon"=w305:string)  [unwired: 1 in]
            n181 = Match Pattern(string=w305, regular expression="ALL-ICONS" ("string")) -> (after substring=w302:string, offset past match=w303:i32)  [unwired: 1 in, 2 out]
            n182 = case shown="-1" w303 {
              tunnel: w305 -> [_ w311]
              tunnel: w302 -> [w307 _]
              tunnel: ["Idle" "UpdateIconPreview"] -> w301
              frame 0, Default {
                n183 = Spreadsheet String To Array(format string="%s", spreadsheet string=w307, array type (2D Dbl)=string[] []) -> (array=w310:string[])  [unwired: 1 in]
                n184 = property on="_Icon" class="Ring (strict)"("Strings []"=w310) -> ()  [unwired: 2 in, 2 out]
              }
              frame -1 {
                n185 = property on="_Icon" class="Ring (strict)"() -> ("Strings []"=w312:string[])  [unwired: 2 in, 2 out]
                n186 = Search 1D Array(1D array=w312, element=w311) -> (index of element=w314:i32)  [unwired: 1 in]
                n187 = case shown="Default" w314 {
                  selector: w314 -> [_ w319]
                  tunnel: w312 -> [w316 _]
                  tunnel: w311 -> [w317 _]
                  frame Default {
                    n188 = Array Size(array=w316) -> (size(s)=w315:i32)
                    n189 = Build Array (concatenate)(w316, w317) -> (w318:string[])
                    n190 = property on="_Icon" class="Ring (strict)"("Strings []"=w318, "Value"=w315) -> ()  [unwired: 2 in, 2 out]
                  }
                  frame 0.. {
                    n191 = local write "_Icon"(w319) -> ()
                  }
                }
              }
            }
          }
          event "_EdgeThickness", "_CenterThickness": Value Change {
            n192 = event-data() -> ()  [unwired: 1 in, 1 out]
          }
          event "_Help": Value Change {
            n193 = event-data() -> ()  [unwired: 1 in, 1 out]
            n194 = call <resource>:"GOOP_HelpMain.vi"() -> ()  [unwired: 12 in]
          }
          event "_Dice": Value Change {
            n195 = event-data() -> ()  [unwired: 1 in, 1 out]
            n196 = control-ref of="_TunnelsAndTerminalsColors"() -> (w329:refnum<vi>)
            n197 = control-ref of="_EdgeColor"() -> (w327:refnum<vi>)
            n198 = control-ref of="_CenterColor1"() -> (w324:refnum<vi>)
            n199 = control-ref of="_CenterColor2"() -> (w323:refnum<vi>)
            n200 = control-ref of="_CenterPattern"() -> (w328:refnum<vi>)
            n201 = control-ref of="_CenterThickness"() -> (w326:refnum<vi>)
            n202 = control-ref of="_EdgeThickness"() -> (w325:refnum<vi>)
            n203 = call <resource>:"BaseProvider_RandomWireConfig.vi"("EdgeColor"=w327, "_CenterThickness"=w326, "_EdgeThickness"=w325, "_CenterColor2"=w324, "_CenterColor1"=w323, "_CenterPattern"=w328, "_TunnelsAndTerminalsColors"=w329) -> ()  [unwired: 13 in]
            n204 = local write "_Dice"(cluster{"Boolean 2":bool, "Dice":bool} {"Boolean 2"=TRUE, "Dice"=FALSE} ("Dice")) -> ()
          }
          event "WireStyleList": Value Change {
            n205 = event-data() -> ("OldVal"=w331:T2[], "NewVal"=w336:T2[])  [unwired: 1 in, 1 out]
            n206 = for {
              tunnel: w336 -> [w361] mode=indexing
              tunnel: [w360] -> w335 mode=indexing
              n207 = Unbundle By Name(w361) -> ("Boolean"=w360:bool)
            }
            n208 = Search 1D Array(1D array=w335, element=TRUE) -> (index of element=w333:i32)  [unwired: 1 in]
            n209 = case shown="0, Default" w333 {
              selector: w333 -> [w339 _]
              tunnel: [w337 _] -> w332
              tunnel: w331 -> [w342 _]
              frame 0, Default {
                w344 = T4 {"Decal"=FALSE, "Color"=11184810} ("Edge color")
                n210 = call <resource>:"BaseProvider_WireStylesManager.vi"() -> ("AllWireConfigurations"=w359:T8[], "AllWireConfigurations(Names)"=w341:string[])  [unwired: 8 in, 2 out]
                n211 = local write "WireStyleList"(w342) -> ()
                n212 = Index Array(array=w341, index=w339) -> (element=w340:string)
                n213 = Index Array(array=w359, index=w339) -> (element=w343:T8)
                n214 = local write "WireStyleName"(w340) -> ()
                n215 = Unbundle By Name(w343) -> ("Edge thickness"=w346:i32, "Edge color"=w358:u32, "Center thickness"=w349:i32, "Center pattern"=w350:T5, "CenterColor1"=w357:u32, "CenterColor2"=w356:u32, "Tunnels and terminals colors"=w355:u32)
                n216 = Format Into String(format string="UpdateWirePreView\nUpdateWireStyleList>>%d\nUpdate", w339) -> (resulting string=w337:string)  [unwired: 2 in, 1 out]
                n217 = Decrement(x=w349) -> (x-1=w348:i32)
                n218 = Bundle(cluster=w344, "Color"=w358) -> (w351:T4)  [unwired: 1 in]
                n219 = Bundle(cluster=w344, "Color"=w357) -> (w352:T4)  [unwired: 1 in]
                n220 = Bundle(cluster=w344, "Color"=w356) -> (w353:T4)  [unwired: 1 in]
                n221 = Bundle(cluster=w344, "Color"=w355) -> (w354:T4)  [unwired: 1 in]
                n222 = local write "_TunnelsAndTerminalsColors"(w354) -> ()
                n223 = To Unsigned Word Integer(number=w346) -> (unsigned 16bit integer=w345:u16)
                n224 = To Unsigned Word Integer(number=w348) -> (unsigned 16bit integer=w347:u16)
                n225 = local write "_CenterThickness"(w347) -> ()
                n226 = local write "_EdgeThickness"(w345) -> ()
                n227 = local write "_CenterPattern"(w350) -> ()
                n228 = local write "_CenterColor1"(w352) -> ()
                n229 = local write "_CenterColor2"(w353) -> ()
                n230 = local write "_EdgeColor"(w351) -> ()
              }
              frame -1 {
              }
            }
          }
          event "WireStyleName": Value Change {
            n231 = event-data() -> ()  [unwired: 1 in, 6 out]
          }
          event "DiscardChanges": Value Change {
            n232 = event-data() -> ()  [unwired: 1 in, 1 out]
            n233 = local read "WireStyleName"() -> (w368:string)
            n234 = call <resource>:"BaseProvider_WireStylesManager.vi"() -> ("AllWireConfigurations"=w365:T8[], "AllWireConfigurations(Names)"=w367:string[])  [unwired: 8 in, 2 out]
            n235 = call <vilib>:"Trim Whitespace.vi"("string"=w368) -> ("trimmed string"=w366:string)  [unwired: 1 in]
            n236 = Search 1D Array(1D array=w367, element=w366) -> (index of element=w364:i32)  [unwired: 1 in]
            n237 = case shown="0, Default" w364 {
              selector: w364 -> [w386 _]
              tunnel: w365 -> [w387 _]
              tunnel: ["UpdateWirePreView\nUpdate" _] -> w363
              frame 0, Default {
                w371 = T4 {"Decal"=FALSE, "Color"=11184810} ("Edge color")
                n238 = Index Array(array=w387, index=w386) -> (element=w370:T8)
                n239 = Unbundle By Name(w370) -> ("Edge thickness"=w373:i32, "Edge color"=w385:u32, "Center thickness"=w376:i32, "Center pattern"=w377:T5, "CenterColor1"=w384:u32, "CenterColor2"=w383:u32, "Tunnels and terminals colors"=w382:u32)
                n240 = Decrement(x=w376) -> (x-1=w375:i32)
                n241 = Bundle(cluster=w371, "Color"=w385) -> (w378:T4)  [unwired: 1 in]
                n242 = Bundle(cluster=w371, "Color"=w384) -> (w379:T4)  [unwired: 1 in]
                n243 = Bundle(cluster=w371, "Color"=w383) -> (w380:T4)  [unwired: 1 in]
                n244 = Bundle(cluster=w371, "Color"=w382) -> (w381:T4)  [unwired: 1 in]
                n245 = local write "_TunnelsAndTerminalsColors"(w381) -> ()
                n246 = To Unsigned Word Integer(number=w373) -> (unsigned 16bit integer=w372:u16)
                n247 = To Unsigned Word Integer(number=w375) -> (unsigned 16bit integer=w374:u16)
                n248 = local write "_CenterThickness"(w374) -> ()
                n249 = local write "_EdgeThickness"(w372) -> ()
                n250 = local write "_CenterPattern"(w377) -> ()
                n251 = local write "_CenterColor1"(w379) -> ()
                n252 = local write "_CenterColor2"(w380) -> ()
                n253 = local write "_EdgeColor"(w378) -> ()
              }
              frame -1 {
              }
            }
          }
          event "DeleteWireStyle": Value Change {
            n254 = event-data() -> ()  [unwired: 1 in, 6 out]
            n255 = local read "WireStyleList"() -> (w391:T2[])
            n256 = for {
              tunnel: w391 -> [w398] mode=indexing
              tunnel: [w396] -> w390
              tunnel: [w395] -> _
              tunnel: [w394] -> w389
              i -> [w395]
              stop <- w394 stop-if-true
              n257 = Unbundle By Name(w398) -> ("Name"=w396:string, "Status"=w397:u16)
              n258 = Not Equal To 0?(x=w397) -> (x != 0?=w394:bool)
            }
            n259 = case shown="True" w389 {
              tunnel: w390 -> [_ w392]
              frame False {
              }
              frame True {
                n260 = call <resource>:"BaseProvider_WireStylesManager.vi"("Action(Read)"=enum16{"Read", "UpdateOne", "DeleteOne"}."DeleteOne", "WireStyleName(Default)"=w392) -> ()  [unwired: 6 in, 4 out]
              }
            }
          }
          event "Update/AddWireStyle": Value Change {
            n261 = event-data() -> ()  [unwired: 1 in, 6 out]
            n262 = Unbundle By Name(w403) -> ("CurrentWireStyle"=w402:T8)
            n263 = local read "WireStyleName"() -> (w400:string)
            n264 = call <resource>:"BaseProvider_WireStylesManager.vi"("Action(Read)"=enum16{"Read", "UpdateOne", "DeleteOne"}."UpdateOne", "WireConfiguration(New or Updating)"=w402, "WireStyleName(Default)"=w400) -> ()  [unwired: 5 in, 4 out]
          }
          event "Up", "Down": Value Change {
            n265 = event-data() -> ()  [unwired: 1 in, 6 out]
            n266 = local read "WireStyleList"() -> (w414:T2[])
            n267 = Unbundle By Name(w417) -> ("CurrentWireStyle"=w416:T8)
            n268 = for {
              tunnel: w414 -> [w422] mode=indexing
              tunnel: [w419] -> w405
              tunnel: [w418] -> w412
              i -> [w418]
              stop <- w420 stop-if-true
              n269 = Unbundle By Name(w422) -> ("Name"=w419:string, "Status"=w421:u16)
              n270 = Not Equal To 0?(x=w421) -> (x != 0?=w420:bool)
            }
            n271 = Increment(x=w412) -> (x+1=w413:i32)
            n272 = Decrement(x=w412) -> (x-1=w411:i32)
            n273 = Select(t=w413, s="Down", f=w411) -> (s? t:f=w407:i32)
            n274 = call <resource>:"BaseProvider_WireStylesManager.vi"("Action(Read)"=enum16{"Read", "UpdateOne", "DeleteOne"}."UpdateOne", "NewIndex(-1=NoChange/Inserted Last If not found)"=w407, "WireConfiguration(New or Updating)"=w416, "WireStyleName(Default)"=w405) -> ("AllWireConfigurations(Names)"=w406:string[])  [unwired: 4 in, 3 out]
            n275 = Search 1D Array(1D array=w406, element=w405) -> (index of element=w404:i32)  [unwired: 1 in]
            n276 = Format Into String(format string="UpdateWirePreView\nUpdateWireStyleList>>%d\nUpdate", w404) -> (resulting string=w408:string)  [unwired: 2 in, 1 out]
          }
          event "_Dice": Mouse Enter {
            n277 = event-data() -> ()  [unwired: 1 in, 1 out]
            n278 = local write "_Dice"(cluster{"Boolean 2":bool, "Dice":bool} {"Boolean 2"=TRUE, "Dice"=FALSE} ("Dice")) -> ()
          }
          event "_Dice": Mouse Leave {
            n279 = event-data() -> ()  [unwired: 1 in, 1 out]
            n280 = local write "_Dice"(cluster{"Boolean 2":bool, "Dice":bool} {"Boolean 2"=FALSE, "Dice"=FALSE} ("Dice")) -> ()
          }
          event "_HelpDefaultConfiguration": Value Change {
            n281 = event-data() -> ()  [unwired: 1 in, 1 out]
            n282 = fn#1354() -> (1:w428:bool)  [unwired: 1 out]
            n283 = Not(x=w428) -> (.not. x?=w427:bool)
            n284 = Control Help Window(1:w427) -> ()  [unwired: 1 in]
          }
        }
      }
      frame "UpdateClass" {
        n285 = local read "_CenterColor1"() -> (w451:T4)
        n286 = local read "_CenterColor2"() -> (w455:T4)
        n287 = local read "_EdgeColor"() -> (w453:T4)
        n288 = local read "_CenterThickness"() -> (w452:T6)
        n289 = local read "_EdgeThickness"() -> (w457:T7)
        n290 = local read "_TunnelsAndTerminalsColors"() -> (w450:T4)
        n291 = local read "_CenterPattern"() -> (w460:T5)
        n292 = Format Into String("_DefaultConnectorPanePattern") -> (resulting string=w433:string)  [unwired: 3 in, 1 out]
        n293 = Unbundle By Name(w465) -> ("ClassRefCreated"=w467:bool, "ClassRef"=w432:refnum<vi>)
        n294 = disable-structure shown="Enabled" {
          disable-tunnel: [w476 _] -> w445
          frame Enabled {
            n295 = property on="_Icon" class="Ring (strict)"() -> ("Strings []"=w478:string[])  [unwired: 2 in, 2 out]
            n296 = local read "_Icon"() -> (w477:u16)
            n297 = Index Array(array=w478, index=w477) -> (element=w476:string)
          }
          frame Disabled {
          }
        }
        n298 = To Unsigned Long Integer(number=w452) -> (unsigned 32bit integer=w454:u32)
        n299 = Unbundle(w451) -> ("Color"=w461:u32)  [unwired: 1 out]
        n300 = Unbundle(w455) -> ("Color"=w462:u32)  [unwired: 1 out]
        n301 = Unbundle(w450) -> ("Color"=w463:u32)  [unwired: 1 out]
        n302 = Unbundle(w453) -> ("Color"=w458:u32)  [unwired: 1 out]
        n303 = Increment(x=w454) -> (x+1=w459:u32)
        n304 = call <resource>:"GDSLvClass_ReadClassType.vi"("Class Refnum In"=w432, "error in (no error)"=w437) -> ("Class Refnum Out"=w439:refnum<vi>, "ClassSettings"=w436:T13, "error out"=w440:errorcluster)  [unwired: 15 in]
        n305 = Bundle By Name(cluster=w436, "ConnectorPanePattern"=w433) -> (w435:T13)
        n306 = call <resource>:"GDSLvClass_StoreClassType.vi"("Class Refnum In"=w439, "ClassSettings"=w435, "error in (no error)"=w440) -> ("Class Refnum Out"=w431:refnum<vi>, "error out"=w438:errorcluster)  [unwired: 15 in]
        n307 = Bundle(cluster=T8 {"Edge thickness"=0, "Edge color"=0, "Center thickness"=0, "Center pattern"=enum."Solid", "CenterColor1"=0, "CenterColor2"=0, "Tunnels and terminals colors"=0} ("WireConfiguration"), "Edge thickness"=w457, "Edge color"=w458, "Center thickness"=w459, "Center pattern"=w460, "CenterColor1"=w461, "CenterColor2"=w462, "Tunnels and terminals colors"=w463) -> (w449:T8)
        n308 = disable-structure shown="Enabled" {
          disable-tunnel: w445 -> [w474 _]
          disable-tunnel: [w471 w475] -> w430
          disable-tunnel: w438 -> [w473 w475]
          disable-tunnel: w431 -> [w472 _]
          frame Enabled {
            n309 = call <resource>:"GDSLvClass_StoreClassItemIcon.vi"("Library Refnum"=w472, "ClassItemIconName"=w474, "error in (no error)"=w473) -> ("error out"=w471:errorcluster)  [unwired: 15 in, 1 out]
          }
          frame Disabled {
          }
        }
        n310 = call <resource>:"GOOP_WirePenTranslator.vi"("WireConfigurationIn"=w449) -> ("WirePensOut"=w464:T16)  [unwired: 17 in, 1 out]
        n311 = property class="LVClassLibrary"(reference=w431, error in=w430, "Wire Pens"=w464) -> (reference out=w448:refnum<vi>, error out=w447:errorcluster)
        n312 = invoke class="LVClassLibrary" method="Save"(reference=w448, error in=w447) -> (reference out=w446:refnum<vi>, error out=w442:errorcluster)  [unwired: 2 in, 2 out]
        n313 = case shown="True" w467 {
          tunnel: w442 -> [w482 w485]
          tunnel: w446 -> [_ w484]
          tunnel: [w482 w483] -> w441
          frame False {
          }
          frame True {
            n314 = Close Reference(reference=w484, error in (no error)=w485) -> (error out=w483:errorcluster)
          }
        }
        n315 = Unbundle By Name(w441) -> ("code"=w444:i32)
        n316 = case shown="Default" w444 {
          tunnel: w437 -> [w479 _]
          tunnel: [w479 w481] -> w443
          tunnel: w441 -> [_ w481]
          frame 8 {
            n317 = One Button Dialog(message="Warning\nThe changes could not be saved.\nThe file might be read-only.") -> ()  [unwired: 1 in, 1 out]
          }
          frame Default {
          }
        }
        n318 = Select(t="SaveConfiguration", s="_SetToDefaultForAllClasses", f="Exit") -> (s? t:f=w470:string)
      }
      frame "UpdateIconPreview" {
        n319 = property on="_Icon" class="Ring (strict)"() -> ("Strings []"=w489:string[])  [unwired: 2 in, 2 out]
        n320 = local read "_Icon"() -> (w488:u16)
        n321 = Index Array(array=w489, index=w488) -> (element=w487:string)
        n322 = call <resource>:"GOOP_GetOverlayIconPath.vi"("IconName(NoPngExtension)"=w487) -> ("IconPath"=w486:path)  [unwired: 10 in]
        n323 = Empty String/Path?(string/path=w486) -> (empty?=w490:bool)
        n324 = case shown="False" w490 {
          tunnel: w486 -> [w494 _]
          frame False {
            n325 = call <vilib>:"Read PNG File.vi"("path to PNG file"=w494) -> ("image data"=w497:T18)  [unwired: 8 in, 2 out]
            n326 = call <resource>:"GOOP_DrawWirePreview_ZoomImage.vi"("image data 2"=w497, "Zoom"=5) -> ("image data"=w498:T18)
            n327 = call <vilib>:"Draw Flattened Pixmap.vi"("image data"=w498) -> ("new picture"=→"_Preview":picture)  [unwired: 8 in]
          }
          frame True {
          }
        }
      }
      frame "SaveConfiguration" {
        n328 = local read "_CenterColor1"() -> (w520:T4)
        n329 = local read "_CenterColor2"() -> (w519:T4)
        n330 = local read "_EdgeColor"() -> (w523:T4)
        n331 = local read "_CenterThickness"() -> (w522:T6)
        n332 = local read "_EdgeThickness"() -> (w524:T7)
        n333 = local read "_TunnelsAndTerminalsColors"() -> (w518:T4)
        n334 = local read "_CenterPattern"() -> (w521:T5)
        n335 = local read "_DefaultConnectorPanePattern"() -> (w513:T3)
        n336 = property on="_Icon" class="Ring (strict)"() -> ("Strings []"=w510:string[])  [unwired: 2 in, 2 out]
        n337 = local read "_Icon"() -> (w511:u16)
        n338 = Index Array(array=w510, index=w511) -> (element=w509:string)
        n339 = To Unsigned Long Integer(number=w522) -> (unsigned 32bit integer=w531:u32)
        n340 = case shown="True" w512 {
          tunnel: [w532 w538] -> w508
          tunnel: w509 -> [w532 w533]
          frame False {
          }
          frame True {
            n341 = call <resource>:"BaseProvider_IniFileSettings.vi"() -> ("IniFileSettings"=w536:T12, "error out"=w534:errorcluster)  [unwired: 18 in]
            n342 = Bundle By Name(cluster=w536, "InterfaceIcon"=w533) -> (w537:T12)
            n343 = call <resource>:"BaseProvider_ConfigurationMemory.vi"() -> ("IconOut"=w538:string)  [unwired: 13 in, 6 out]
            n344 = call <resource>:"BaseProvider_IniFileSettings.vi"("IniFileSettings"=w537, "error in (no error)"=w534, "Action"=enum16{"Read", "Load", "Save"}."Save") -> ()  [unwired: 15 in, 2 out]
          }
        }
        n345 = Increment(x=w531) -> (x+1=w530:u32)
        n346 = Unbundle(w520) -> ("Color"=w528:u32)  [unwired: 1 out]
        n347 = Unbundle(w519) -> ("Color"=w529:u32)  [unwired: 1 out]
        n348 = Unbundle(w518) -> ("Color"=w526:u32)  [unwired: 1 out]
        n349 = Unbundle(w523) -> ("Color"=w527:u32)  [unwired: 1 out]
        n350 = Bundle By Name(cluster=T8 {"Edge thickness"=0, "Edge color"=0, "Center thickness"=0, "Center pattern"=enum."Solid", "CenterColor1"=0, "CenterColor2"=0, "Tunnels and terminals colors"=0} ("WireConfiguration"), "Edge thickness"=w524, "Edge color"=w527, "Center thickness"=w530, "Center pattern"=w521, "CenterColor1"=w528, "CenterColor2"=w529, "Tunnels and terminals colors"=w526) -> (w502:T8)
        n351 = call <resource>:"BaseProvider_WireStylesManager.vi"() -> ("AllWireConfigurations"=w503:T8[])  [unwired: 8 in, 3 out]
        n352 = Bundle By Name(cluster=T10 {"FlatFolderStructure"=FALSE, "CleanUpBDForPropertyMethods"=FALSE} ("OptionsIn"), "FlatFolderStructure"="_FlatFolderStructure", "CleanUpBDForPropertyMethods"="_CleanUpBDForPropertyMethods") -> (w507:T10)
        n353 = call <resource>:"BaseProvider_ConfigurationMemory.vi"("WireConfiguration"=w502, "Icon"=w508, "Action"=enum16{"Read", "Load", "Save"}."Save", "PatternIn"=w513) -> ()  [unwired: 9 in, 7 out]
        n354 = Search 1D Array(1D array=w503, element=w502) -> (index of element=w500:i32)  [unwired: 1 in]
        n355 = Bundle By Name(cluster=w515, "SelectedWireStyleIndex"=w500) -> (w501:T9)
        n356 = call <resource>:"GOOP400_ConfigurationMemory.vi"("OptionsIn"=w507, "Action"=enum16{"Read", "Load", "Save"}."Save") -> ()  [unwired: 16 in, 2 out]
      }
    }
  }
  "Error Out" <- w27
  n357 = disable-structure shown="Disabled" {
    frame Disabled {
      n358 = property on="_EdgeThickness" class="Enum (strict)"("Val(Sgnl)"=T7."1 pixel" ("Value (Signaling)")) -> ()  [unwired: 2 in, 2 out]
    }
    frame Enabled {
    }
  }
  n359 = Generate User Event(user event=w25, event data cluster="Stop" ("Stop")) -> (user event out=w26:refnum<user-event>)  [unwired: 2 in, 1 out]
  n360 = Destroy User Event(user event=w26) -> (error out=w14:errorcluster)  [unwired: 1 in]
  n361 = Destroy User Event(user event=w12, error in=w14) -> (error out=w13:errorcluster)
  n362 = case shown="False" w11 {
    tunnel: [CommonVIs_ClassIconSelection_Action."All" ("IconsToShow(All)") CommonVIs_ClassIconSelection_Action."Only Interface" ("IconsToShow(All)")] -> w4
    frame False {
    }
    frame True {
    }
  }
  n363 = Unregister For Events(event registration refnum=w15, error in=w13) -> ()  [unwired: 1 out]
  n364 = control-ref of="IconSelection"() -> (w2:refnum<vi>)
  n365 = control-ref of="Icon"() -> (w3:refnum<vi>)
  n366 = call <resource>:"CommonVIs_ClassIconSelection.vi"("SaveChangesInClassRightAway(True)"=FALSE, "IconSelected"=w12, "IconsToShow(All)"=w4, "Icon"=w3, "error in (no error)"=w10, "Messages(Stop or Empty string will stop this VI)"=w20, "IconSelection"=w2, "LVClassToActOn"=w17) -> ()  [unwired: 4 in]
  n367 = call <resource>:"GDSString_AddStatesToQueue.vi"() -> ()  [unwired: 15 in, 1 out]
  n368 = Unbundle By Name(w6) -> ("SelectedWireStyleIndex"=→"SelectedWireStyleIndex":i32)
